vi "CRYSet Curve Library Front Panel.vi"(11 "Vi Ref In":refnum<vi> caption="Vi Ref") -> (3 "Vi Ref Out":refnum<vi> caption="Vi Ref")   [LabVIEW 2013]
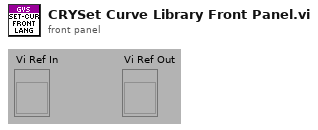
[diagram p1: front panel]
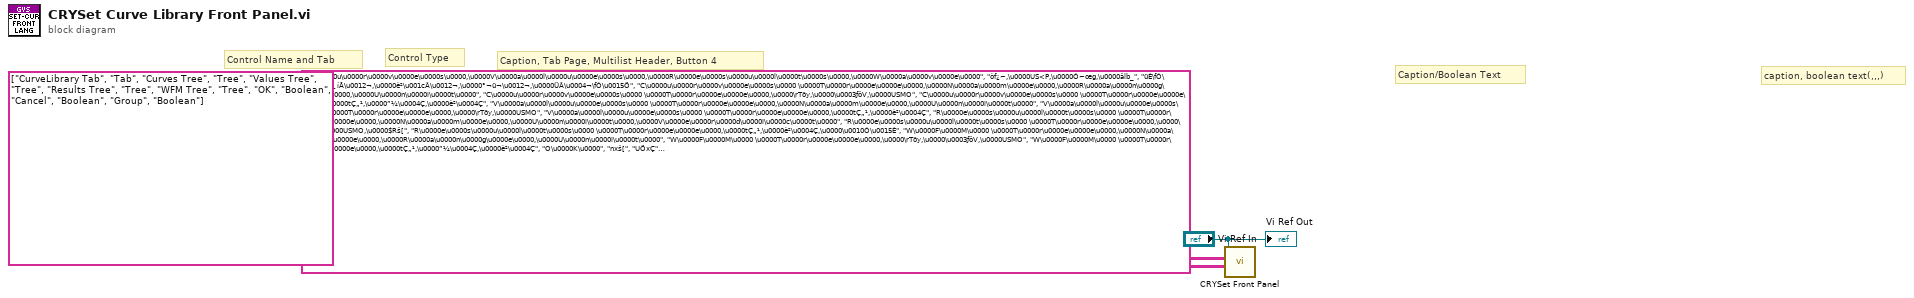
[diagram p0: block diagram]
diagram:
  # "Caption, Tab Page, Multilist Header, Button 4"
  # "Control Type"
  # "Control Name and Tab"
  # "caption, boolean text(,,,)"
  # "Caption/Boolean Text"
  n1 = call "CRYSet Front Panel.vi"("Caption(Boolean Text)"=string[][] [["C\u0000u\u0000r\u0000v\u0000e\u0000s\u0000,\u0000V\u0000a\u0000l\u0000u\u0000e\u0000s\u0000,\u0000R\u0000e\u0000s\u0000u\u0000l\u0000t\u0000s\u0000,\u0000W\u0000a\u0000v\u0000e\u0000", "òf¿~,\u0000US<P,\u0000Ó~œg,\u0000âlb_", "üÈ\fÓ\u0018Â9¸íÅ\u0012¬,\u0000è²\u001cÂ\u0012¬,\u0000°¬ü¬\u0012¬,\u0000ÜÂ\u0004¬\fÓ\u0015Ö"], ["C\u0000u\u0000r\u0000v\u0000e\u0000s\u0000 \u0000T\u0000r\u0000e\u0000e\u0000,\u0000N\u0000a\u0000m\u0000e\u0000,\u0000R\u0000a\u0000n\u0000g\u0000e\u0000,\u0000U\u0000n\u0000i\u0000t\u0000", "C\u0000u\u0000r\u0000v\u0000e\u0000s\u0000 \u0000T\u0000r\u0000e\u0000e\u0000,\u0000\rTðy,\u0000\u0003ƒôV,\u0000USMO", "C\u0000u\u0000r\u0000v\u0000e\u0000s\u0000 \u0000T\u0000r\u0000e\u0000e\u0000,\u0000tÇ„¹,\u0000”¼\u0004Ç,\u0000è²\u0004Ç"], ["V\u0000a\u0000l\u0000u\u0000e\u0000s\u0000 \u0000T\u0000r\u0000e\u0000e\u0000,\u0000N\u0000a\u0000m\u0000e\u0000,\u0000U\u0000n\u0000i\u0000t\u0000", "V\u0000a\u0000l\u0000u\u0000e\u0000s\u0000 \u0000T\u0000r\u0000e\u0000e\u0000,\u0000\rTðy,\u0000USMO", "V\u0000a\u0000l\u0000u\u0000e\u0000s\u0000 \u0000T\u0000r\u0000e\u0000e\u0000,\u0000tÇ„¹,\u0000è²\u0004Ç"], ["R\u0000e\u0000s\u0000u\u0000l\u0000t\u0000s\u0000 \u0000T\u0000r\u0000e\u0000e\u0000,\u0000N\u0000a\u0000m\u0000e\u0000,\u0000U\u0000n\u0000i\u0000t\u0000,\u0000V\u0000e\u0000r\u0000d\u0000i\u0000c\u0000t\u0000", "R\u0000e\u0000s\u0000u\u0000l\u0000t\u0000s\u0000 \u0000T\u0000r\u0000e\u0000e\u0000,\u0000\rTðy,\u0000USMO,\u0000$Rš[", "R\u0000e\u0000s\u0000u\u0000l\u0000t\u0000s\u0000 \u0000T\u0000r\u0000e\u0000e\u0000,\u0000tÇ„¹,\u0000è²\u0004Ç,\u0000\u0010Ó\u0015È"], ["W\u0000F\u0000M\u0000 \u0000T\u0000r\u0000e\u0000e\u0000,\u0000N\u0000a\u0000m\u0000e\u0000,\u0000R\u0000a\u0000n\u0000g\u0000e\u0000,\u0000U\u0000n\u0000i\u0000t\u0000", "W\u0000F\u0000M\u0000 \u0000T\u0000r\u0000e\u0000e\u0000,\u0000\rTðy,\u0000\u0003ƒôV,\u0000USMO", "W\u0000F\u0000M\u0000 \u0000T\u0000r\u0000e\u0000e\u0000,\u0000tÇ„¹,\u0000”¼\u0004Ç,\u0000è²\u0004Ç"], ["O\u0000K\u0000", "nxš[", "UÖxÇ"], ["C\u0000a\u0000n\u0000c\u0000e\u0000l\u0000", "ÖSˆm", "èÍŒÁ"], ["G\u0000r\u0000o\u0000u\u0000p\u0000 \u0000S\u0000e\u0000l\u0000e\u0000c\u0000t\u0000e\u0000d\u0000 \u0000I\u0000t\u0000e\u0000m\u0000s\u0000", "ûm R@b\tyîv0R\u0000N*N°evÄ~", " ÁÝÐ\\Õ \u0000mÕ©ºä´DÇ \u0000ÈÀø­ù¸ÐÅ \u0000”Í\u0000¬"]], "Control ID and Type(Label Name, Type)"=string[][] [["CurveLibrary Tab", "Tab"], ["Curves Tree", "Tree"], ["Values Tree", "Tree"], ["Results Tree", "Tree"], ["WFM Tree", "Tree"], ["OK", "Boolean"], ["Cancel", "Boolean"], ["Group", "Boolean"]], "Vi Ref"="Vi Ref In") -> ()  [unwired: 9 in]
  "Vi Ref Out" <- "Vi Ref In"
